vi "Calculate Intervals.vi"(8 "gap/group ratio":dbl, 9 "Num Intervals":i32, 10 "End":refnum<class "Vec3d Class.lvclass">, 11 "Start":refnum<class "Vec3d Class.lvclass">) -> (2 "Intervals":T1[](array[typedef]))   [LabVIEW 2011]
uses:
  Vec3d Class/Vec3d Class.lvclass
  Type Definitions/3d Line.ctl
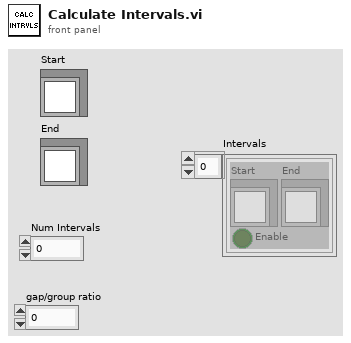
[diagram p1: front panel]
types:
  T1 = typedef "3d Line.ctl" = cluster{"Start":refnum<class "Vec3d Class.lvclass">, "End":refnum<class "Vec3d Class.lvclass">, "Enable":bool}
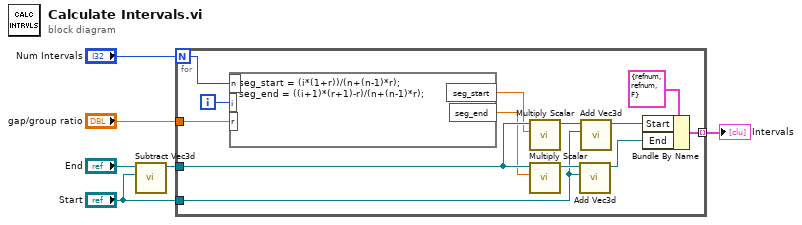
[diagram p0: block diagram]
diagram:
  n1 = call "Subtract Vec3d.vi"("Vec3d in 2"="Start", "Vec3d in 1"="End") -> ("Vec3d Class out"=w5:refnum<class "Vec3d Class.lvclass">)  [unwired: 8 in, 1 out]
  n2 = for {
    N: "Num Intervals" -> [w19]
    tunnel: w5 -> [w16]
    tunnel: "gap/group ratio" -> [w17]
    tunnel: "Start" -> [w11]
    tunnel: [w7] -> w1 mode=indexing
    i -> [w18]
    n3 = formula code="seg_start = (i*(1+r))/(n+(n-1)*r);\nseg_end = ((i+1)*(r+1)-r)/(n+(n-1)*r);"("n"=w19, "i"=w18, "r"=w17) -> ("seg_start"=w15:dbl, "seg_end"=w14:dbl)
    n4 = call-dynamic "Multiply Scalar.vi"("Scale"=w15, "Vec3d in"=w16) -> ("Vec3d out"=w13:refnum<class "Vec3d Class.lvclass">)  [unwired: 8 in, 1 out]
    n5 = call-dynamic "Multiply Scalar.vi"("Scale"=w14, "Vec3d in"=w16) -> ("Vec3d out"=w12:refnum<class "Vec3d Class.lvclass">)  [unwired: 8 in, 1 out]
    n6 = call-dynamic "Add Vec3d.vi"(10:"Vec3d Class in"=w11, 11:"Vec3d Class in"=w12) -> ("Vec3d Class out"=w8:refnum<class "Vec3d Class.lvclass">)  [unwired: 8 in, 1 out]
    n7 = call-dynamic "Add Vec3d.vi"(10:"Vec3d Class in"=w11, 11:"Vec3d Class in"=w13) -> ("Vec3d Class out"=w9:refnum<class "Vec3d Class.lvclass">)  [unwired: 8 in, 1 out]
    n8 = Bundle By Name(cluster=T1 {"Start"=refnum, "End"=refnum, "Enable"=FALSE} ("Potting Line"), "Start"=w9, "End"=w8) -> (w7:T1)
  }
  "Intervals" <- w1
